vi "GBD_Header.vi"(7 "Head":string, 8 "Save?":bool, 9 "Mode":enum16{"Open", "Close", "Index"}(ring), 10 "Cvt_Mode":bool, 11 "File[]":path[](array[path])) -> (0 "error out":errorcluster, 1 "ActiveCH":i32, 2 "List":string[][](array[string]), 3 "Param":T1={"File"=[refnum], "Idx"=[], "dT"=0.5, "Hd"=4096, "Rd"=14, "Start"=[timestamp(3519879471 s since 1904-01-01)], "Trig"=[timestamp(3519879472 s since 1904-01-01)], "Stop"=[timestamp(3519940623 s since 1904-01-01)], "FirstPos"=[], "Count"=[120609], "Color"=[27836, 4765252, 11010216, 14712848], "Label"=["CH1", "CH2", "CH3", "CH4"], "INP"=["CH1", "CH2", "CH3", "CH4"], "H"=[5.0, 5.0, 5.0, 5.0], "L"=[-5.0, -5.0, -5.0, -5.0], "Fmt"=["%.;%+0.3f V", "%.;%+0.3f V", "%.;%+0.3f V", "%.;%+0.3f V"], "Unit"=["", "", "", ""], "SEL"=[0, 1, 2, 3], "Byte"=[-2, -2, -2, -2], "Pos"=[], "Bit"=[], "Flg"=[], "Gain"=[], "Offset"=[0.01, 0.01, 0.01, 0.01], "CH"=[0, 0, 0, 0], "Opt"={"Mode"=0, "TUNIT"=enum."CELS"}, "TYPE"=enum."GBD", "Comp"=[], "Temp"=[]} caption="HEAD" {"FirstPos" format="%<%x %.3X>T"; "Stop" format="%<%x %.3X>T"; "Trig" format="%<%x %.3X>T"; "Start" format="%<%x %.3X>T"}, 4 "Linkcheck":string[](array[string])=["Sampling", "Start", "Trigger", "Stop", "Count"])   [LabVIEW 2017]
uses:
  Amp_Param.ctl
panel:
  in  "Info":string[](array[string])=["Sampling", "Start", "Trigger", "Stop", "Count"]
  # "ALL"
  # "GBD"
  # "CSV"
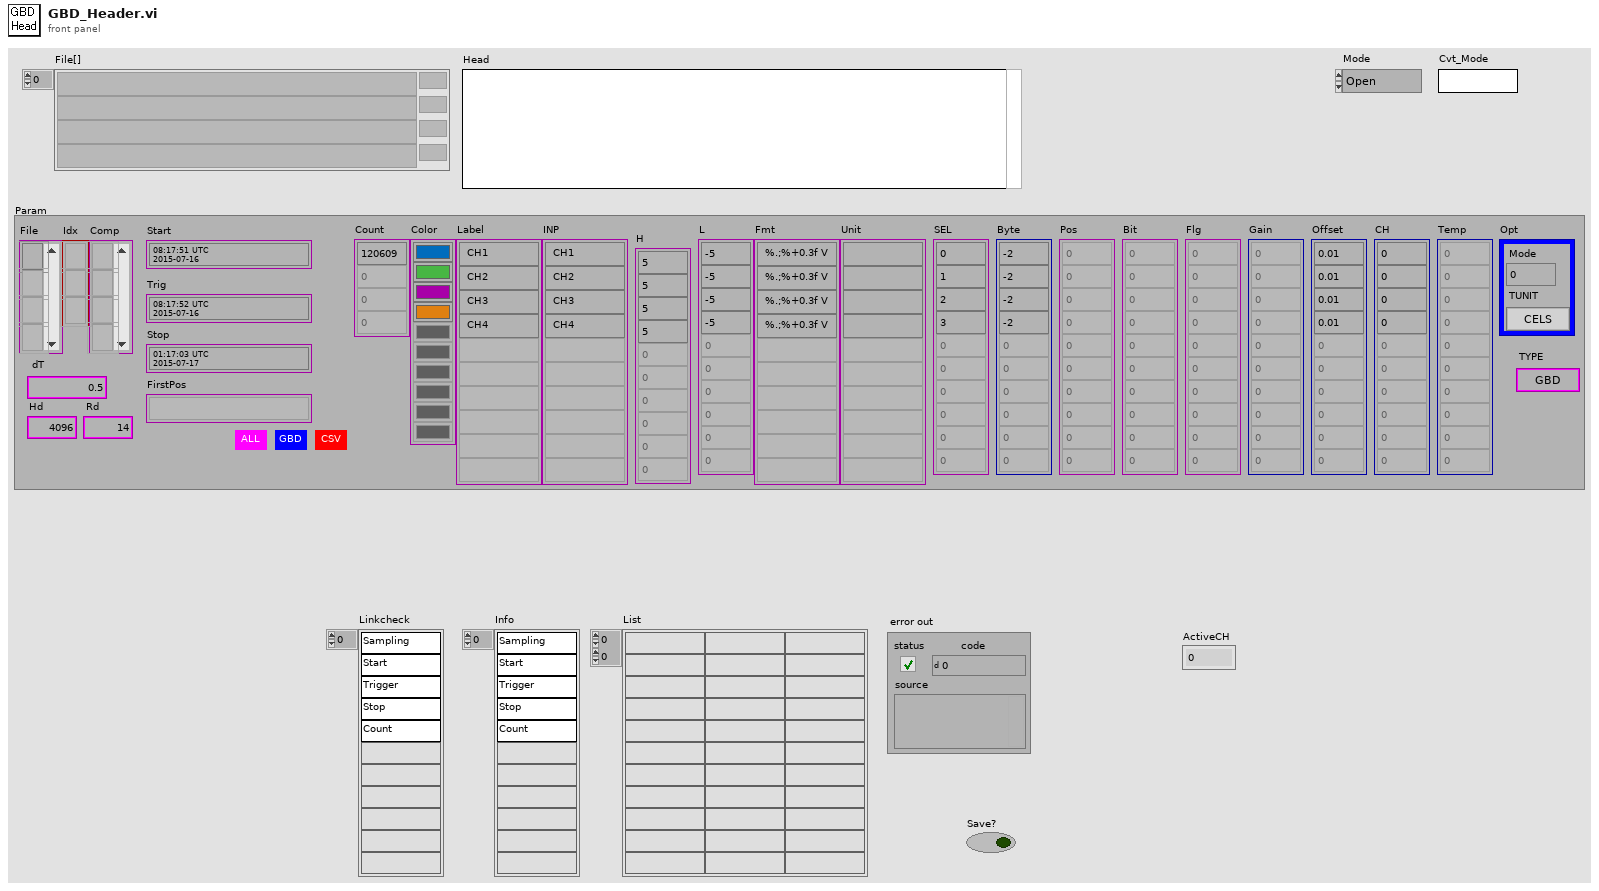
[diagram p1: front panel]
types:
  T1 = typedef "Amp_Param.ctl" = cluster{"File":refnum<file>[], "Idx":refnum<file>[], "dT":dbl, "Hd":i32, "Rd":i32, "Start":timestamp[], "Trig":timestamp[], "Stop":timestamp[], "FirstPos":timestamp[], "Count":i64[], "Color":u32[], "Label":string[], "INP":string[], "H":dbl[], "L":dbl[], "Fmt":string[], "Unit":string[], "SEL":i32[], "Byte":i32[], "Pos":i32[], "Bit":i32[], "Flg":i32[], "Gain":dbl[], "Offset":dbl[], "CH":i32[], "Opt":cluster{"Mode":i32, "TUNIT":enum16{"CELS", "FAHR"}}, "TYPE":enum16{"GBD", "CSV"}, "Comp":refnum<file>[], "Temp":i32[]}
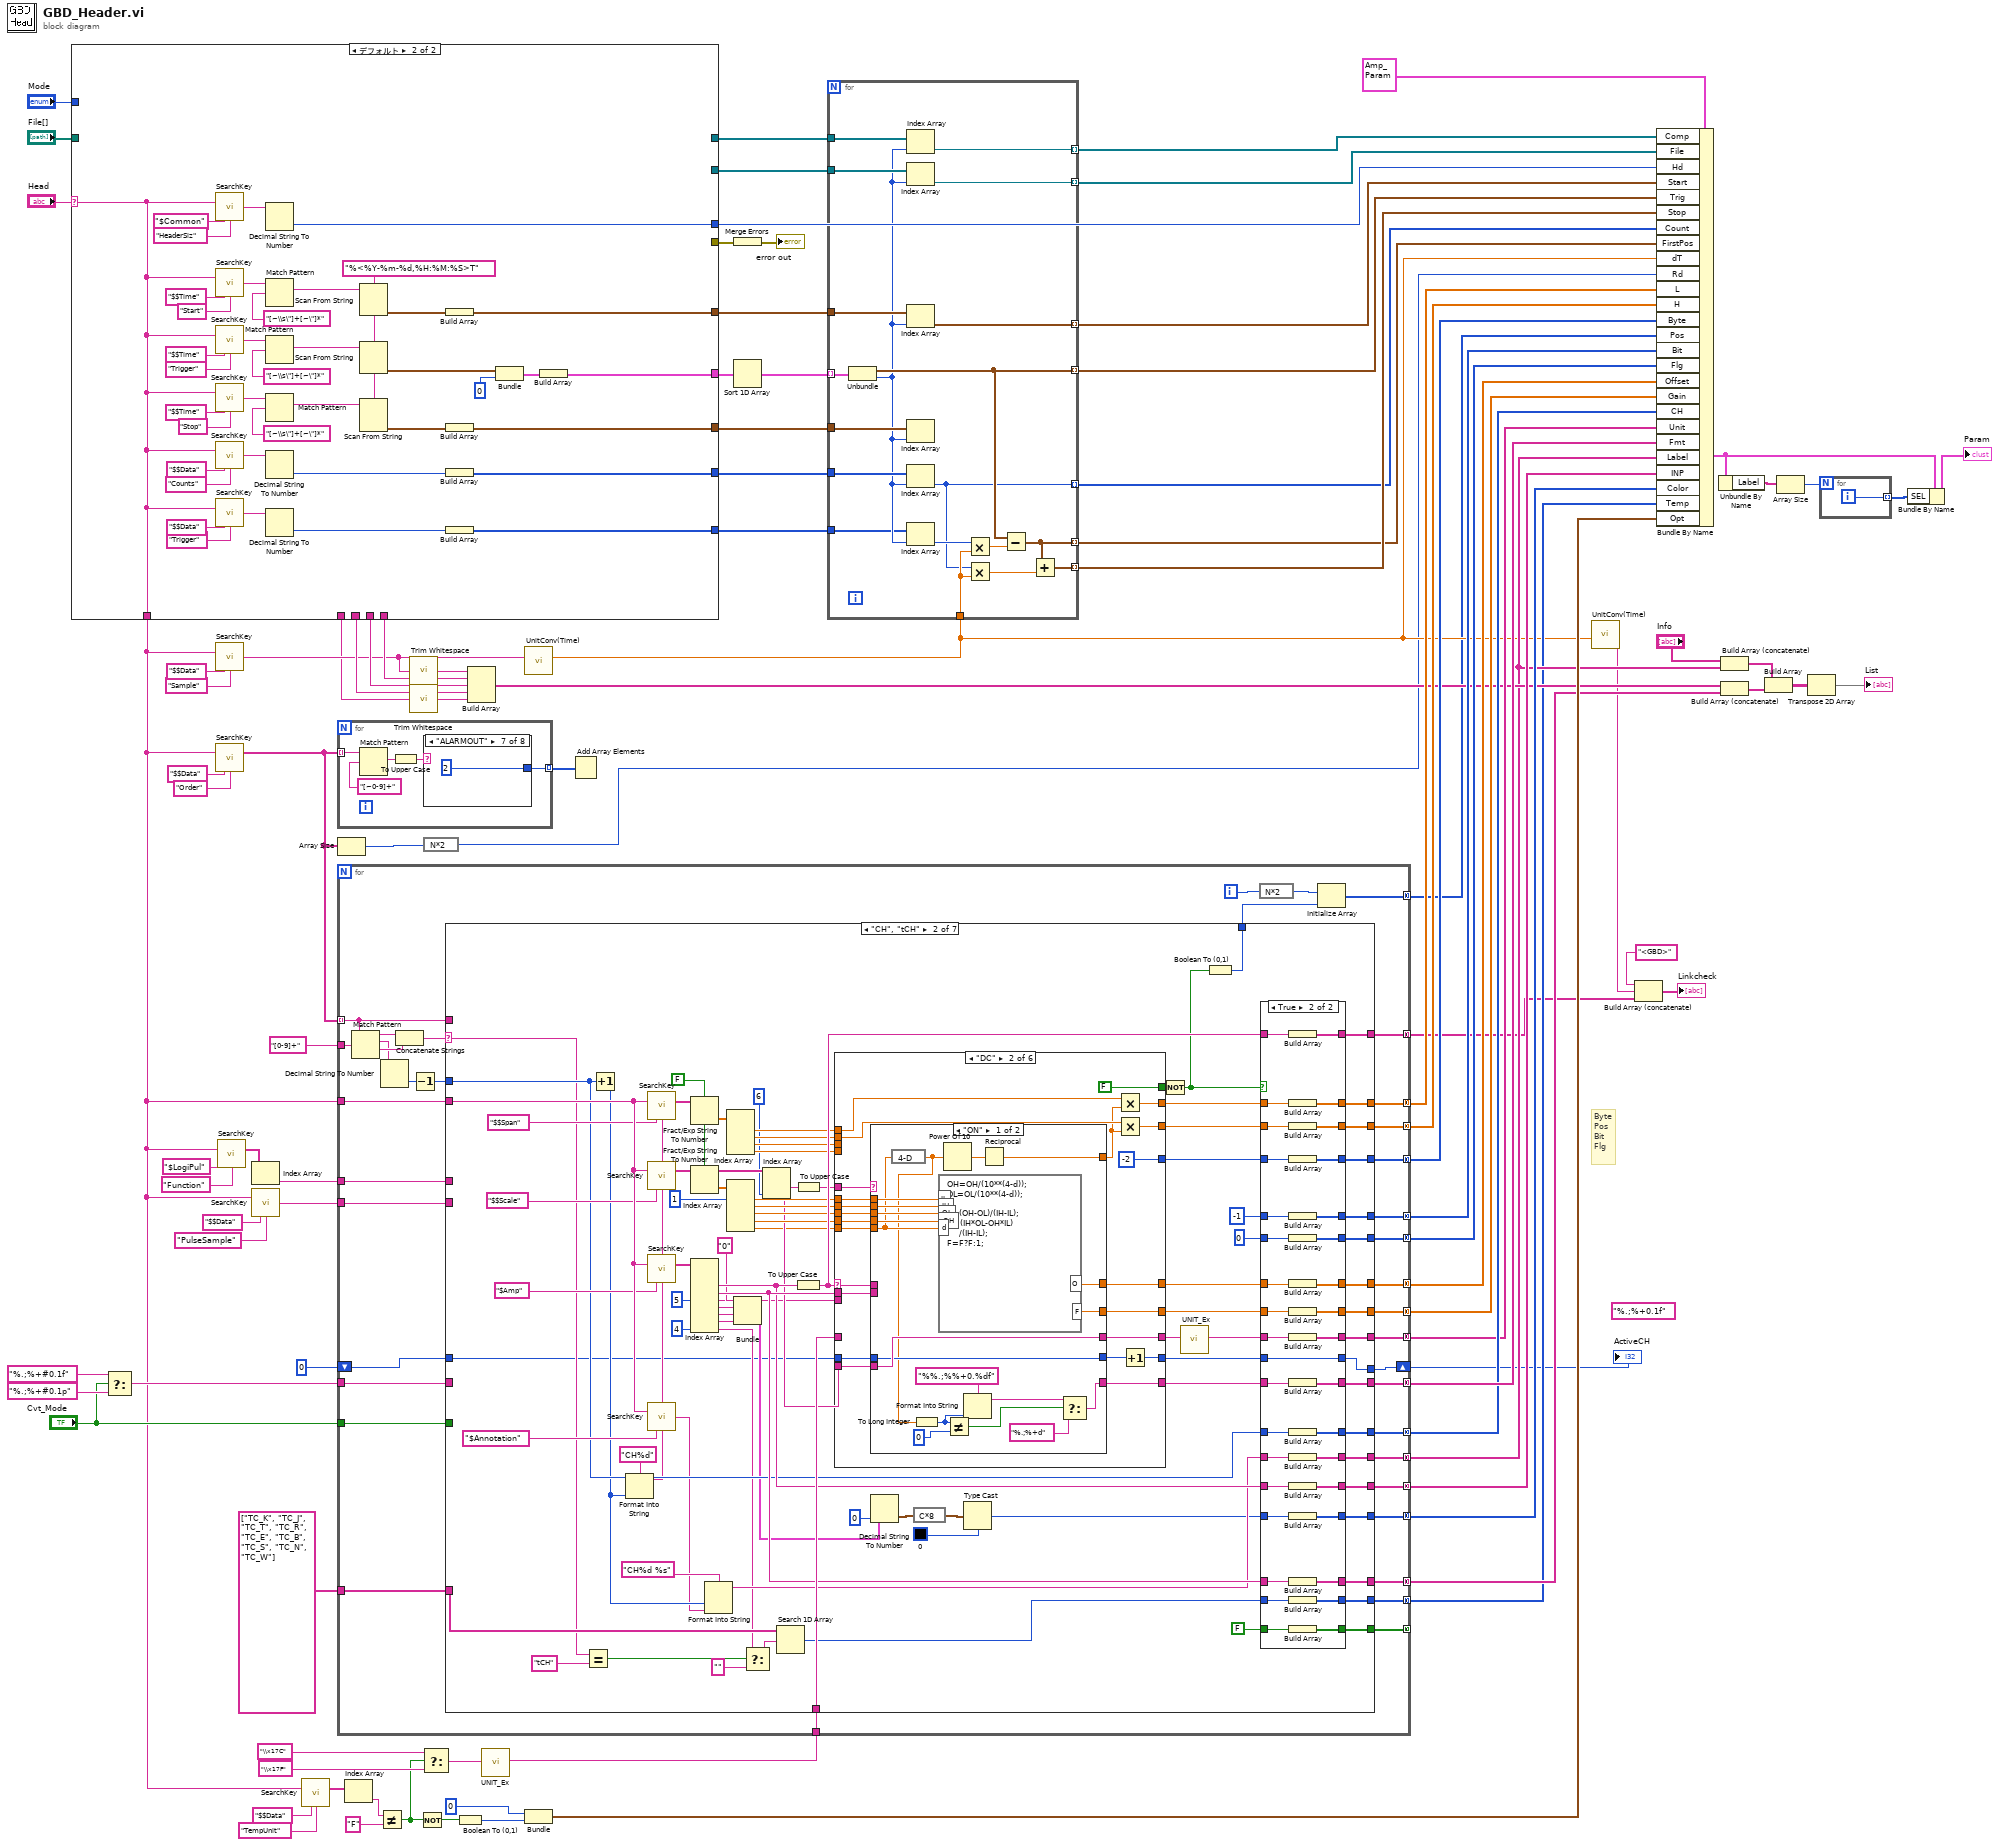
[diagram p0: block diagram]
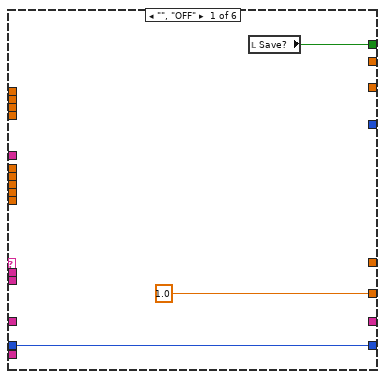
[diagram p4: hidden frame]
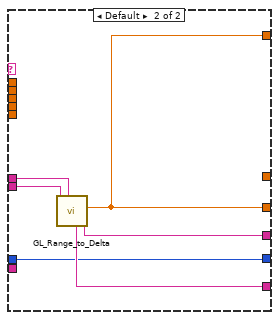
[diagram p5: hidden frame]
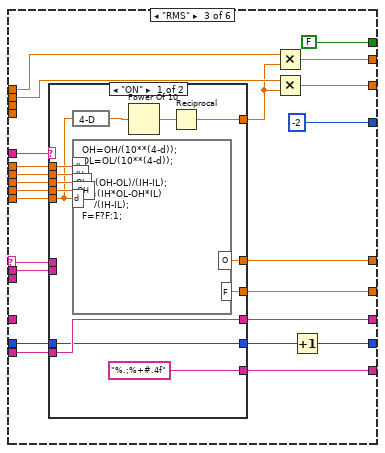
[diagram p6: hidden frame]
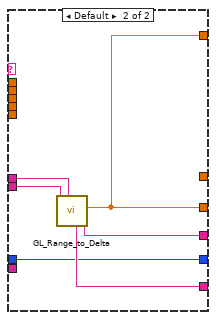
[diagram p7: hidden frame]
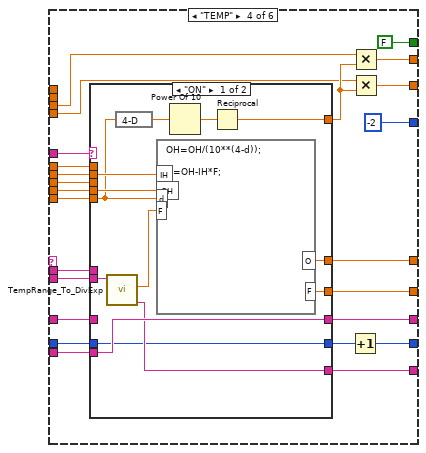
[diagram p8: hidden frame]
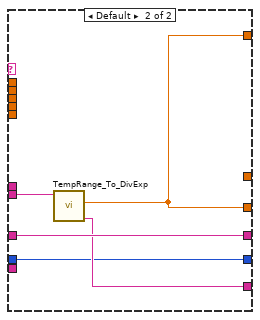
[diagram p9: hidden frame]
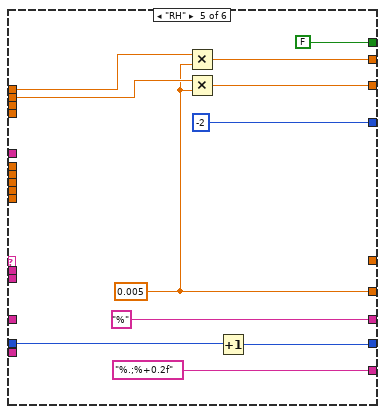
[diagram p10: hidden frame]
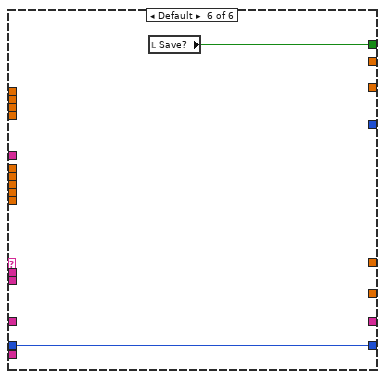
[diagram p11: hidden frame]
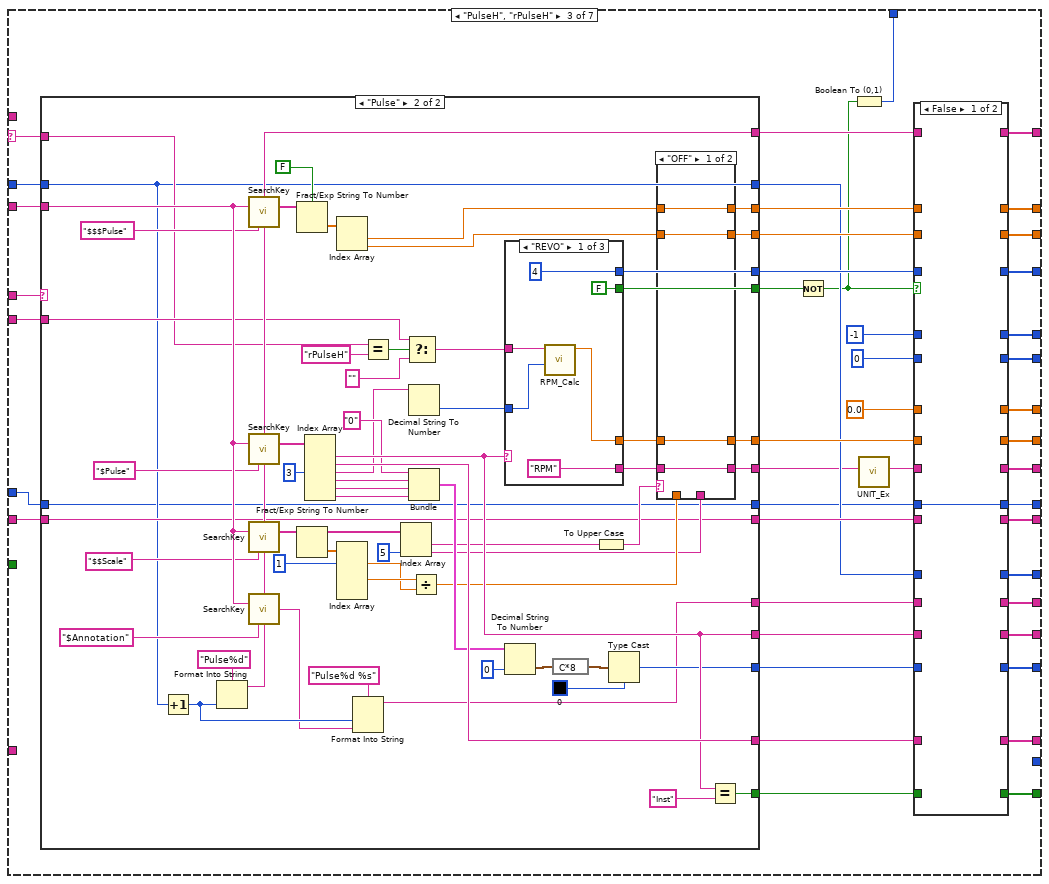
[diagram p12: hidden frame]
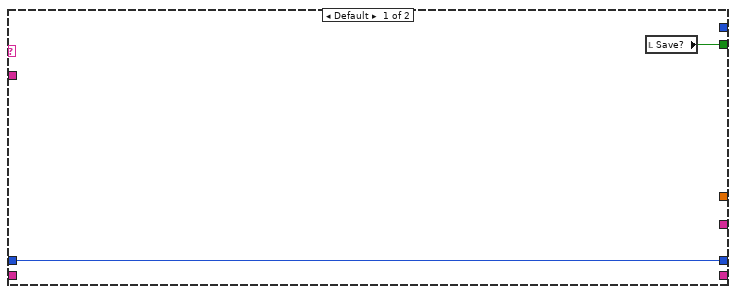
[diagram p13: hidden frame]
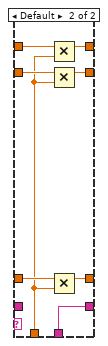
[diagram p14: hidden frame]
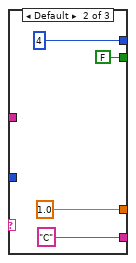
[diagram p15: hidden frame]
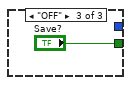
[diagram p16: hidden frame]
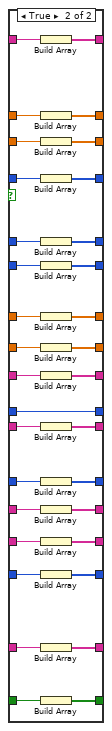
[diagram p17: hidden frame]
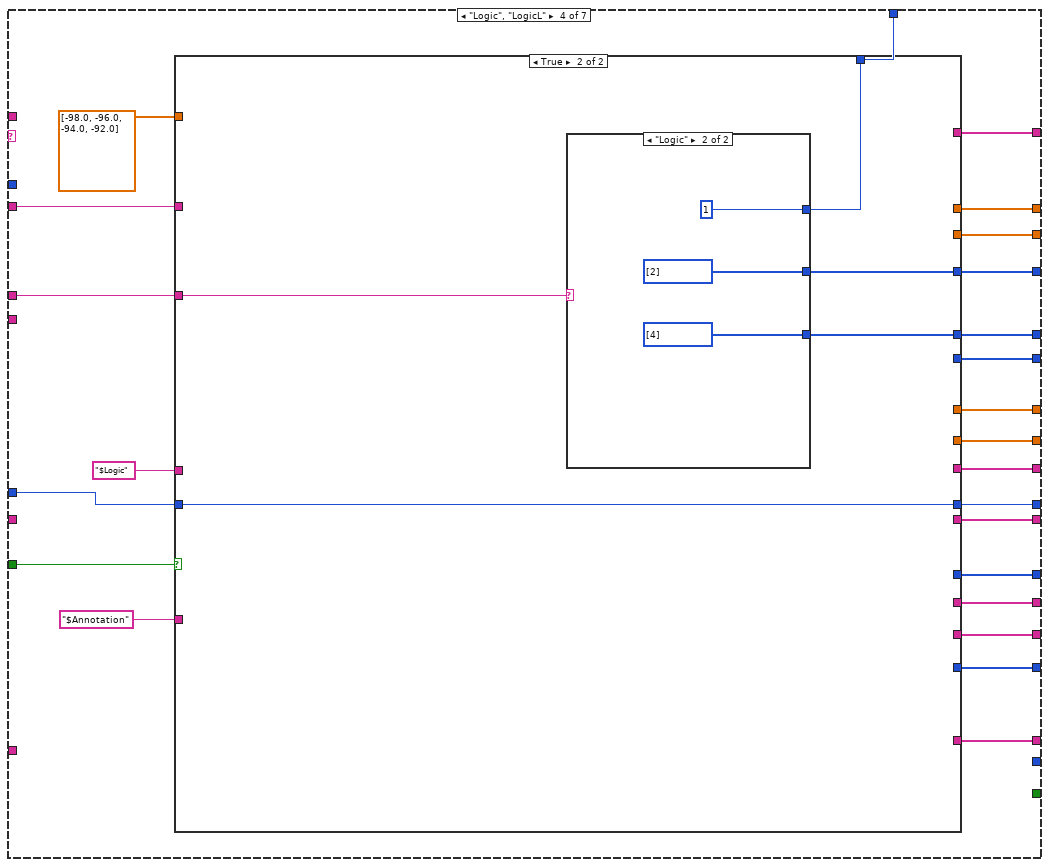
[diagram p18: hidden frame]
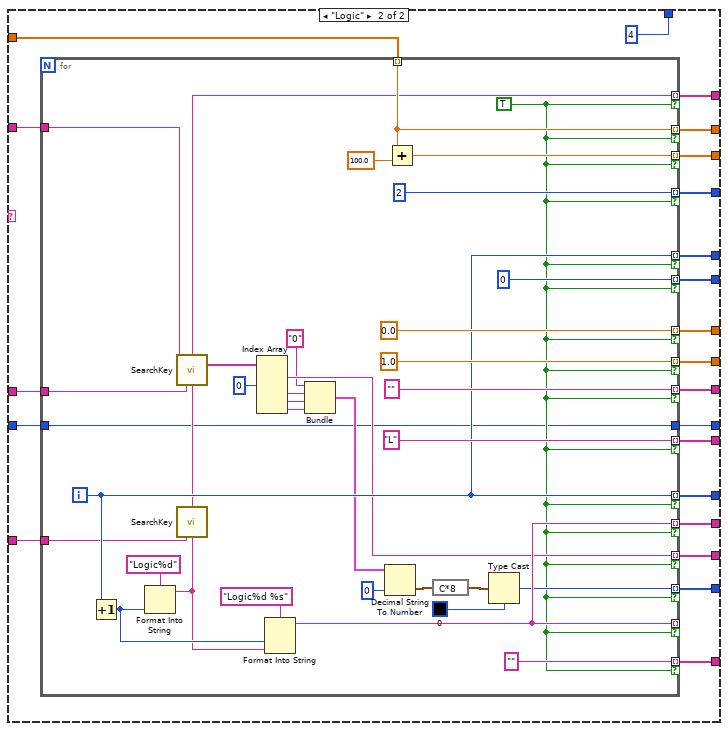
[diagram p20: hidden frame]
diagram:
  (unwired) "%.;%+0.1f" ("format string")
  # "Byte\nPos\nBit\nFlg"
  n1 = case shown="デフォルト" "Head" {
    selector: "Head" -> [_ w172]
    tunnel: [w115 _] -> w70
    tunnel: [w114 w185] -> w96
    tunnel: [w113 w172] -> w7
    tunnel: [w111 w209] -> w68
    tunnel: "File[]" -> [w112 _]
    tunnel: [w109 w182] -> w71
    tunnel: [w110 w181] -> w69
    tunnel: [w108 _] -> w77
    tunnel: [w107 _] -> w29
    tunnel: [w106 _] -> w76
    tunnel: "Mode" -> [w105 _]
    tunnel: [w104 w177] -> w74
    tunnel: [w103 _] -> w61
    tunnel: [w102 _] -> w39
    tunnel: [w101 w171] -> w27
    tunnel: [w100 _] -> w20
    frame "" {
      n2 = for {
        tunnel: [w121] -> w113
        tunnel: w112 -> [w130] mode=indexing
        tunnel: [w135] -> w115 mode=indexing
        tunnel: [w128] -> w114
        tunnel: [w148] -> w111 mode=indexing
        tunnel: [w139] -> w110 mode=indexing
        tunnel: [w138] -> w109 mode=indexing
        tunnel: [w125] -> w108
        tunnel: [w124] -> w107
        tunnel: [w126] -> w106
        tunnel: w105 -> [w134]
        tunnel: [w132] -> w104 mode=indexing
        tunnel: [w129] -> w103 mode=indexing
        tunnel: [w127] -> w102
        tunnel: [w120] -> w101 mode=indexing
        tunnel: [w117] -> w100 mode=indexing
        i -> [w133]
        w137 = "%<%Y-%m-%d,%H:%M:%S>T" ("format string")
        n3 = Open/Create/Replace File(file path (use dialog)=w130) -> (refnum out=w156:refnum<file>, error out=w155:errorcluster)  [unwired: 1 in, 5 out]
        n4 = Read from Binary File(8:w155, 10:1024 ("count"), 11:w156) -> (0:w116:errorcluster, 2:w118:string, 3:w162:refnum<file>)  [unwired: 4 out]
        n5 = call "SearchKey.vi"("In"=w118, "KEY1"="$Common", "KEY2"="HeaderSiz") -> ("String"=w159:string)  [unwired: 12 out]
        n6 = Set File Position(refnum=w162, from (0:start)=enum16{"start", "end", "current"}."start" ("pos mode (0:2)"), error in=w116) -> (refnum out=w158:refnum<file>, error out=w157:errorcluster)  [unwired: 1 out]
        n7 = Decimal String To Number(string=w159) -> (number=w128:i32)  [unwired: 3 out]
        n8 = Read from Binary File(8:w157, 10:w128, 11:w158) -> (0:w117:errorcluster, 2:w121:string, 3:w136:refnum<file>)  [unwired: 4 out]
        n9 = call "SearchKey.vi"("In"=w121, "KEY1"="$$Time", "KEY2"="Start") -> ("String"=w147:string)  [unwired: 12 out]
        n10 = call "SearchKey.vi"("In"=w121, "KEY1"="$$Time", "KEY2"="Trigger") -> ("String"=w149:string)  [unwired: 12 out]
        n11 = call "SearchKey.vi"("In"=w121, "KEY1"="$$Time", "KEY2"="Stop") -> ("String"=w140:string)  [unwired: 12 out]
        n12 = call "SearchKey.vi"("In"=w121, "KEY1"="$$Data", "KEY2"="Counts") -> ("String"=w124:string)  [unwired: 12 out]
        n13 = call "SearchKey.vi"("In"=w121, "KEY1"="$$Data", "KEY2"="Trigger") -> ("String"=w123:string)  [unwired: 12 out]
        n14 = Match Pattern(string=w147, regular expression="[~\\s\"]+[~\"]*") -> (match substring=w127:string)  [unwired: 4 out]
        n15 = Match Pattern(string=w149, regular expression="[~\\s\"]+[~\"]*") -> (match substring=w126:string)  [unwired: 4 out]
        n16 = Match Pattern(string=w140, regular expression="[~\\s\"]+[~\"]*") -> (match substring=w125:string)  [unwired: 4 out]
        n17 = Decimal String To Number(string=w123) -> (number=w120:i32)  [unwired: 3 out]
        n18 = Scan From String(format string=w137, input string=w127) -> (output 1=w138:timestamp)  [unwired: 3 in, 3 out]
        n19 = Scan From String(format string=w137, input string=w126) -> (output 1=w131:timestamp)  [unwired: 3 in, 3 out]
        n20 = Scan From String(format string=w137, input string=w125) -> (output 1=w139:timestamp)  [unwired: 3 in, 3 out]
        n21 = Decimal String To Number(string=w124) -> (number=w148:i32)  [unwired: 3 out]
        n22 = case shown="デフォルト" w134 {
          tunnel: w136 -> [w165 w170]
          tunnel: [_ w170] -> w135
          tunnel: w130 -> [_ w169]
          tunnel: [_ w167] -> w129
          tunnel: w128 -> [_ w166]
          frame "Close" {
            n23 = Close File(refnum=w165) -> ()  [unwired: 1 in, 2 out]
          }
          frame Default {
            n24 = Open/Create/Replace File(file path (use dialog)=w169) -> (refnum out=w168:refnum<file>)  [unwired: 1 in, 6 out]
            n25 = Set File Position(offset (in bytes) (0)=w166, refnum=w168) -> (refnum out=w167:refnum<file>)  [unwired: 2 in, 1 out]
          }
        }
        n26 = Bundle(w131, w133) -> (w132:cluster{timestamp, i32})  [unwired: 1 in]
      }
    }
    frame Default {
      w186 = "%<%Y-%m-%d,%H:%M:%S>T" ("format string")
      n27 = call "SearchKey.vi"("In"=w172, "KEY1"="$Common", "KEY2"="HeaderSiz") -> ("String"=w206:string)  [unwired: 12 out]
      n28 = call "SearchKey.vi"("In"=w172, "KEY1"="$$Time", "KEY2"="Start") -> ("String"=w196:string)  [unwired: 12 out]
      n29 = call "SearchKey.vi"("In"=w172, "KEY1"="$$Time", "KEY2"="Trigger") -> ("String"=w199:string)  [unwired: 12 out]
      n30 = call "SearchKey.vi"("In"=w172, "KEY1"="$$Time", "KEY2"="Stop") -> ("String"=w189:string)  [unwired: 12 out]
      n31 = call "SearchKey.vi"("In"=w172, "KEY1"="$$Data", "KEY2"="Counts") -> ("String"=w203:string)  [unwired: 12 out]
      n32 = call "SearchKey.vi"("In"=w172, "KEY1"="$$Data", "KEY2"="Trigger") -> ("String"=w175:string)  [unwired: 12 out]
      n33 = Decimal String To Number(string=w206) -> (number=w185:i32)  [unwired: 3 out]
      n34 = Match Pattern(string=w196, regular expression="[~\\s\"]+[~\"]*") -> (match substring=w197:string)  [unwired: 4 out]
      n35 = Match Pattern(string=w199, regular expression="[~\\s\"]+[~\"]*") -> (match substring=w198:string)  [unwired: 4 out]
      n36 = Match Pattern(string=w189, regular expression="[~\\s\"]+[~\"]*") -> (match substring=w188:string)  [unwired: 4 out]
      n37 = Decimal String To Number(string=w203) -> (number=w187:i32)  [unwired: 3 out]
      n38 = Decimal String To Number(string=w175) -> (number=w176:i32)  [unwired: 3 out]
      n39 = Scan From String(format string=w186, input string=w197) -> (output 1=w183:timestamp)  [unwired: 3 in, 3 out]
      n40 = Scan From String(format string=w186, input string=w198) -> (output 1=w180:timestamp)  [unwired: 3 in, 3 out]
      n41 = Scan From String(format string=w186, input string=w188) -> (output 1=w184:timestamp)  [unwired: 3 in, 3 out]
      n42 = Build Array(w183) -> (w182:timestamp[])
      n43 = Build Array(w184) -> (w181:timestamp[])
      n44 = Build Array(w187) -> (w209:i32[])
      n45 = Build Array(w176) -> (w171:i32[])
      n46 = Bundle(w180, 0) -> (w179:cluster{timestamp, i32})  [unwired: 1 in]
      n47 = Build Array(w179) -> (w177:cluster{timestamp, i32}[])
    }
  }
  n48 = Select(t="%.;%+#0.1f" ("format string"), s="Cvt_Mode", f="%.;%+#0.1p" ("format string")) -> (s? t:f=w23:string)
  n49 = call "SearchKey.vi"("In"=w7, "KEY1"="$$Data", "KEY2"="Sample") -> ("String"=w32:string)  [unwired: 12 out]
  n50 = call "SearchKey.vi"("In"=w7, "KEY1"="$$Data", "KEY2"="Order") -> ("Data"=w11:string[])  [unwired: 12 out]
  n51 = call "SearchKey.vi"("In"=w7, "KEY1"="$LogiPul", "KEY2"="Function") -> ("Data"=w48:string[])  [unwired: 12 out]
  n52 = Index Array(array=w48) -> (element=w4:string)  [unwired: 1 in]
  n53 = call "SearchKey.vi"("In"=w7, "KEY1"="$$Data", "KEY2"="PulseSample") -> ("String"=w12:string)  [unwired: 12 out]
  n54 = call "SearchKey.vi"("In"=w7, "KEY1"="$$Data", "KEY2"="TempUnit") -> ("Data"=w93:string[])  [unwired: 12 out]
  n55 = for {
    tunnel: w11 -> [w214] mode=indexing
    tunnel: [w211] -> w55 mode=indexing
    n56 = Match Pattern(string=w214, regular expression="[~0-9]+") -> (match substring=w213:string)  [unwired: 4 out]
    n57 = To Upper Case(1:w213) -> (0:w212:string)
    n58 = case shown="\"ALARMOUT\"" w212 {
      tunnel: [_ 2 ("element") 4 ("element") 2 ("element") 2 ("element") 2 ("element") 2 ("element") 2 ("element")] -> w211
      frame Default {
      }
      frame "CH" {
      }
      frame "HCH" {
      }
      frame "LOGIC" {
      }
      frame "ALARM" {
      }
      frame "ALARMLP" {
      }
      frame "ALARMOUT" {
      }
      frame "PULSE" {
      }
    }
  }
  n59 = Array Size(array=w11) -> (size(s)=w10:i32)
  n60 = Index Array(array=w93) -> (element=w87:string)  [unwired: 1 in]
  n61 = Not Equal?(x=w87, y="F") -> (x != y?=w59:bool)
  n62 = call <vilib>:"Trim Whitespace.vi"("string"=w32) -> ("trimmed string"=w31:string)  [unwired: 1 in]
  n63 = call <vilib>:"Trim Whitespace.vi"("string"=w29) -> ("trimmed string"=w30:string)  [unwired: 1 in]
  n64 = Not(x=w59) -> (.not. x?=w86:bool)
  n65 = Select(t="\\x17C" ("y"), s=w59, f="\\x17F" ("y")) -> (s? t:f=w84:string)
  n66 = expression code="N*2"(w10) -> (w9:i32)
  n67 = Boolean To (0,1)(Boolean=w86) -> (0, 1=w85:i16)
  n68 = Build Array(w31, w39, w76, w77, w30) -> (w41:string[])
  n69 = call "UNIT_Ex.vi"("In"=w84) -> ("Out"=w83:string)  [unwired: 10 out]
  n70 = for {
    tunnel: w7 -> [w259]
    tunnel: w83 -> [w258]
    tunnel: [w257] -> w54 mode=concatenating
    tunnel: [w256] -> w53 mode=concatenating
    tunnel: [w255] -> w81 mode=concatenating
    tunnel: [w254] -> w80 mode=concatenating
    tunnel: [w253] -> w79 mode=concatenating
    tunnel: [w252] -> w78 mode=concatenating
    tunnel: [w251] -> w37 mode=concatenating
    tunnel: [w250] -> w40 mode=concatenating
    tunnel: [w249] -> w63 mode=concatenating
    tunnel: [w248] -> w58 mode=concatenating
    tunnel: [w247] -> w57 mode=concatenating
    tunnel: [w246] -> w56 mode=concatenating
    tunnel: [w245] -> w51 mode=concatenating
    tunnel: [w244] -> w47 mode=concatenating
    tunnel: "Cvt_Mode" -> [w243]
    tunnel: [w242] -> w26 mode=concatenating
    tunnel: w23 -> [w241]
    tunnel: [w240] -> _ mode=concatenating
    tunnel: [w239] -> w18 mode=concatenating
    tunnel: w12 -> [w238]
    tunnel: w11 -> [w237] mode=indexing
    tunnel: "[0-9]+" ("KEY2") -> [w236]
    tunnel: [w227] -> w5 mode=concatenating
    tunnel: w4 -> [w230]
    tunnel: string[] ["TC_K", "TC_J", "TC_T", "TC_R", "TC_E", "TC_B", "TC_S", "TC_N", "TC_W"] ("1D array") -> [w225]
    shift-right: [w222] -> w2
    shift-left: 0 -> [w223]
    i -> [w224]
    n71 = Match Pattern(string=w237, regular expression=w236) -> (before substring=w235:string, match substring=w232:string, after substring=w233:string)  [unwired: 1 in, 1 out]
    n72 = Decimal String To Number(string=w232) -> (number=w231:i32)  [unwired: 2 in, 1 out]
    n73 = Concatenate Strings(w235, w233) -> (w234:string)
    n74 = Decrement(x=w231) -> (x-1=w229:i32)
    n75 = case shown="\"CH\", \"tCH\"" w234 {
      selector: w234 -> [_ w269 w553 _ _ _ _]
      tunnel: w259 -> [_ w351 w580 w710 w819 w860 _]
      tunnel: w258 -> [_ w350 _ _ _ _ _]
      tunnel: [_ w294 w566 w724 _ _ _] -> w257
      tunnel: [_ w293 w552 w723 _ _ _] -> w256
      tunnel: [_ w292 w565 w722 w817 w857 w920] -> w255
      tunnel: [_ w289 w562 w721 w822 w863 w919] -> w254
      tunnel: [_ w288 w561 w720 w821 w862 w918] -> w253
      tunnel: [_ w286 w559 w719 _ _ _] -> w252
      tunnel: [_ w284 w550 w718 _ _ _] -> w251
      tunnel: [_ w281 w555 w717 _ _ _] -> w250
      tunnel: [_ w283 w557 w716 _ _ _] -> w249
      tunnel: [_ w285 w558 w714 _ _ _] -> w248
      tunnel: [_ w282 w556 w713 _ _ _] -> w247
      tunnel: [_ w287 w560 w712 _ _ _] -> w246
      tunnel: [_ w291 w564 w711 w820 w861 w917] -> w245
      tunnel: [_ w290 w563 w709 w818 w859 w916] -> w244
      tunnel: w243 -> [_ _ _ w703 w815 w855 w914]
      tunnel: [_ w280 _ _ _ _ _] -> w242
      tunnel: w241 -> [_ _ w547 _ _ _ _]
      tunnel: [_ w279 w554 _ _ _ _] -> w240
      tunnel: [_ w295 w567 w706 _ _ _] -> w239
      tunnel: w238 -> [_ _ w568 _ _ _ _]
      tunnel: w237 -> [_ _ _ _ _ _ _]
      tunnel: w229 -> [_ w331 w545 _ _ _ _]
      tunnel: w230 -> [_ _ w543 w704 _ w858 _]
      tunnel: [_ w276 w541 w705 w816 w856 w915] -> w226
      tunnel: w225 -> [_ w275 _ _ _ _ _]
      tunnel: w223 -> [w260 w263 w538 w702 w814 w854 w913]
      tunnel: [w260 w261 w536 w701 w813 w854 w913] -> w222
      frame Default {
      }
      frame "CH", "tCH" {
        w296 = FALSE ("use system decimal point (T)")
        n76 = Equal?(x=w269, y="tCH") -> (x = y?=w268:bool)
        n77 = Increment(x=w331) -> (x+1=w321:i32)
        n78 = Format Into String(format string="CH%d" ("KEY1"), w321) -> (resulting string=w305:string)  [unwired: 2 in, 1 out]
        n79 = call "SearchKey.vi"("In"=w351, "KEY1"="$$Span", "KEY2"=w305) -> ("Data"=w327:string[])  [unwired: 12 out]
        n80 = call "SearchKey.vi"("In"=w351, "KEY1"="$$Scale", "KEY2"=w305) -> ("Data"=w308:string[])  [unwired: 12 out]
        n81 = call "SearchKey.vi"("In"=w351, "KEY1"="$Amp", "KEY2"=w305) -> ("Data"=w329:string[])  [unwired: 12 out]
        n82 = call "SearchKey.vi"("In"=w351, "KEY1"="$Annotation", "KEY2"=w305) -> ("String"=w320:string)  [unwired: 12 out]
        n83 = Fract/Exp String To Number(use system decimal point (T)=w296, string=w327) -> (number=w326:dbl[])  [unwired: 2 in, 1 out]
        n84 = Fract/Exp String To Number(use system decimal point (T)=w296, string=w308) -> (number=w309:dbl[])  [unwired: 2 in, 1 out]
        n85 = Index Array(array=w329, index #4=5 ("index"), index #8=4 ("index")) -> (element #2=w342:string, element #3=w343:string, element #4=w264:string, element #5=w319:string, element #6=w318:string, element #7=w311:string, element #8=w273:string)  [unwired: 6 in, 1 out]
        n86 = Format Into String(format string="CH%d %s" ("KEY1"), w321, w320) -> (resulting string=w341:string)  [unwired: 2 in, 1 out]
        n87 = Index Array(array=w326) -> (element #1=w325:dbl, element #2=w324:dbl, element #3=w323:dbl, element #4=w322:dbl)  [unwired: 4 in]
        n88 = Index Array(array=w309, index #1=1 ("index")) -> (element #1=w304:dbl, element #2=w303:dbl, element #3=w302:dbl, element #4=w301:dbl, element #5=w298:dbl)  [unwired: 4 in]
        n89 = Bundle("0", w319, w318, w311) -> (w312:cluster{string, string, string, string})  [unwired: 1 in]
        n90 = Select(t=w273, s=w268, f="") -> (s? t:f=w272:string)
        n91 = Index Array(array=w308, index #2=6 ("index")) -> (element #1=w307:string, element #2=w299:string)  [unwired: 1 in]
        n92 = Search 1D Array(1D array=w275, element=w272) -> (index of element=w271:i32)  [unwired: 1 in]
        n93 = To Upper Case(1:w342) -> (0:w332:string)
        n94 = To Upper Case(1:w307) -> (0:w297:string)
        n95 = case shown="\"DC\"" w332 {
          selector: w332 -> [_ w395 w443 _ _ _]
          tunnel: w343 -> [_ w408 w456 w501 _ _]
          tunnel: [1.0 w397 w445 w491 w527 _] -> w345
          tunnel: [_ w407 w455 w485 "%" ("Unit OUT") _] -> w266
          tunnel: w350 -> [_ _ _ w490 _ _]
          tunnel: [_ -2 -2 -2 -2 _] -> w347
          tunnel: w325 -> [_ w409 w457 _ w529 _]
          tunnel: w324 -> [_ w410 w458 _ w528 _]
          tunnel: w323 -> [_ _ _ w488 _ _]
          tunnel: w322 -> [_ _ _ w489 _ _]
          tunnel: [_ w412 w460 w503 w531 _] -> w349
          tunnel: [_ w411 w459 w502 w530 _] -> w348
          tunnel: [_ w406 w454 w500 "%.;%+0.2f" ("format string") _] -> w344
          tunnel: [w389 FALSE ("Save?") FALSE ("Save?") FALSE ("Save?") FALSE ("Save?") w535] -> w278
          tunnel: w304 -> [_ w403 w451 w497 _ _]
          tunnel: w303 -> [_ w402 w450 w496 _ _]
          tunnel: w302 -> [_ w401 w449 w495 _ _]
          tunnel: w301 -> [_ w400 w448 w494 _ _]
          tunnel: w298 -> [_ w399 w447 w493 _ _]
          tunnel: w297 -> [_ w405 w453 w499 _ _]
          tunnel: [_ w404 w452 w498 _ _] -> w346
          tunnel: w299 -> [_ w396 w444 w487 _ _]
          tunnel: w264 -> [_ _ _ w484 _ _]
          tunnel: [w388 w393 w441 w481 w523 w534] -> w262
          tunnel: w263 -> [w388 w391 w439 w483 w524 w534]
          frame "", "OFF" {
            n96 = local read "Save?"() -> (w389:bool)
          }
          frame "DC" {
            n97 = case shown="\"ON\"" w405 {
              tunnel: w408 -> [_ w438]
              tunnel: [w432 w435] -> w397
              tunnel: [w426 w437] -> w407
              tunnel: [w417 w436] -> w406
              tunnel: [w431 _] -> w404
              tunnel: w403 -> [w430 _]
              tunnel: w402 -> [w429 _]
              tunnel: w401 -> [w428 _]
              tunnel: w400 -> [w427 _]
              tunnel: w399 -> [w423 _]
              tunnel: [w424 w435] -> w398
              tunnel: w396 -> [w426 _]
              tunnel: w395 -> [_ w434]
              tunnel: [w422 w433] -> w392
              tunnel: w391 -> [w422 w433]
              frame "ON" {
                n98 = expression code="4-D"(w423) -> (w415:dbl)
                n99 = To Long Integer(number=w415) -> (32bit integer=w414:i32)
                n100 = formula code="OH=OH/(10**(4-d));\nOL=OL/(10**(4-d));\n\nF=(OH-OL)/(IH-IL);\nO=(IH*OL-OH*IL)\n    /(IH-IL);\nF=F?F:1;"("IL"=w430, "IH"=w429, "OL"=w428, "OH"=w427, "d"=w423) -> ("O"=w431:dbl, "F"=w432:dbl)
                n101 = Power Of 10(x=w415) -> (10^x=w425:dbl)
                n102 = Not Equal?(x=w414, y=0) -> (x != y?=w420:bool)
                n103 = Format Into String(format string="%%.;%%+0.%df", w414) -> (resulting string=w419:string)  [unwired: 2 in, 1 out]
                n104 = Reciprocal(x=w425) -> (1/x=w424:dbl)
                n105 = Select(t=w419, s=w420, f="%.;%+d" ("format string")) -> (s? t:f=w417:string)
              }
              frame Default {
                n106 = call "GL_Range_to_Delta.vi"("Input"=w434, "Range"=w438) -> ("Unit"=w437:string, "delta"=w435:dbl, "Fmt"=w436:string)  [unwired: 5 in]
              }
            }
            n107 = Multiply(x=w409, y=w398) -> (x*y=w412:dbl)
            n108 = Multiply(x=w410, y=w398) -> (x*y=w411:dbl)
            n109 = Increment(x=w392) -> (x+1=w393:i32)
          }
          frame "RMS" {
            n110 = case shown="\"ON\"" w453 {
              tunnel: w456 -> [_ w480]
              tunnel: [w474 w477] -> w445
              tunnel: [w467 w479] -> w455
              tunnel: ["%.;%+#.4f" ("Fmt") w478] -> w454
              tunnel: [w473 _] -> w452
              tunnel: w451 -> [w472 _]
              tunnel: w450 -> [w471 _]
              tunnel: w449 -> [w470 _]
              tunnel: w448 -> [w469 _]
              tunnel: w447 -> [w464 _]
              tunnel: [w463 w477] -> w446
              tunnel: w444 -> [w467 _]
              tunnel: w443 -> [_ w476]
              tunnel: [w462 w475] -> w440
              tunnel: w439 -> [w462 w475]
              frame "ON" {
                n111 = expression code="4-D"(w464) -> (w465:dbl)
                n112 = formula code="OH=OH/(10**(4-d));\nOL=OL/(10**(4-d));\n\nF=(OH-OL)/(IH-IL);\nO=(IH*OL-OH*IL)\n    /(IH-IL);\nF=F?F:1;"("IL"=w472, "IH"=w471, "OL"=w470, "OH"=w469, "d"=w464) -> ("O"=w473:dbl, "F"=w474:dbl)
                n113 = Power Of 10(x=w465) -> (10^x=w466:dbl)
                n114 = Reciprocal(x=w466) -> (1/x=w463:dbl)
              }
              frame Default {
                n115 = call "GL_Range_to_Delta.vi"("Input"=w476, "Range"=w480) -> ("Unit"=w479:string, "delta"=w477:dbl, "Fmt"=w478:string)  [unwired: 5 in]
              }
            }
            n116 = Multiply(x=w457, y=w446) -> (x*y=w460:dbl)
            n117 = Multiply(x=w458, y=w446) -> (x*y=w459:dbl)
            n118 = Increment(x=w440) -> (x+1=w441:i32)
          }
          frame "TEMP" {
            n119 = case shown="\"ON\"" w499 {
              tunnel: w501 -> [_ _]
              tunnel: [w517 w520] -> w491
              tunnel: [w511 w522] -> w485
              tunnel: [w506 w519] -> w500
              tunnel: [w516 _] -> w498
              tunnel: w497 -> [_ _]
              tunnel: w496 -> [w514 _]
              tunnel: w495 -> [_ _]
              tunnel: w494 -> [w515 _]
              tunnel: w493 -> [w510 _]
              tunnel: [w512 w520] -> w492
              tunnel: w490 -> [_ w522]
              tunnel: w487 -> [w511 _]
              tunnel: w484 -> [w507 w521]
              tunnel: w483 -> [w505 w518]
              tunnel: [w505 w518] -> w482
              frame "ON" {
                n120 = call "TempRange_To_DivExp.vi"("Range"=w507) -> ("Exp"=w506:string, "Div"=w508:dbl)  [unwired: 8 in]
                n121 = expression code="4-D"(w510) -> (w509:dbl)
                n122 = formula code="OH=OH/(10**(4-d));\n\nO=OH-IH*F;"("IH"=w514, "OH"=w515, "d"=w510, "F"=w508) -> ("O"=w516:dbl, "F"=w517:dbl)
                n123 = Power Of 10(x=w509) -> (10^x=w513:dbl)
                n124 = Reciprocal(x=w513) -> (1/x=w512:dbl)
              }
              frame Default {
                n125 = call "TempRange_To_DivExp.vi"("Range"=w521) -> ("Exp"=w519:string, "Div"=w520:dbl)  [unwired: 8 in]
              }
            }
            n126 = Increment(x=w482) -> (x+1=w481:i32)
            n127 = Multiply(x=w488, y=w492) -> (x*y=w503:dbl)
            n128 = Multiply(x=w489, y=w492) -> (x*y=w502:dbl)
          }
          frame "RH" {
            w527 = 0.005
            n129 = Multiply(x=w529, y=w527) -> (x*y=w531:dbl)
            n130 = Multiply(x=w528, y=w527) -> (x*y=w530:dbl)
            n131 = Increment(x=w524) -> (x+1=w523:i32)
          }
          frame Default {
            n132 = local read "Save?"() -> (w535:bool)
          }
        }
        n133 = Decimal String To Number(string=w312, default (0L)=u8 0 ("index")) -> (number=w315:cluster{u8, u8, u8, u8})  [unwired: 1 in, 1 out]
        n134 = expression code="C*8"(w315) -> (w313:cluster{u8, u8, u8, u8})
        n135 = Type Cast(type=u32 0 ("Color"), x=w313) -> (*(type *) &x=w338:u32)
        n136 = Not(x=w278) -> (.not. x?=w277:bool)
        n137 = call "UNIT_Ex.vi"("In"=w266) -> ("Out"=w265:string)  [unwired: 10 out]
        n138 = Boolean To (0,1)(Boolean=w277) -> (0, 1=w276:i16)
        n139 = case shown="TRUE" w277 {
          tunnel: w349 -> [_ w387]
          tunnel: w348 -> [_ w386]
          tunnel: w347 -> [_ w385]
          tunnel: w346 -> [_ w384]
          tunnel: w345 -> [_ w383]
          tunnel: w344 -> [_ w382]
          tunnel: w343 -> [_ w381]
          tunnel: w342 -> [_ w380]
          tunnel: w341 -> [_ w379]
          tunnel: w338 -> [_ w378]
          tunnel: w265 -> [_ w377]
          tunnel: -1 -> [_ w376]
          tunnel: 0 -> [_ w375]
          tunnel: w271 -> [_ w374]
          tunnel: FALSE -> [_ w373]
          tunnel: w332 -> [_ w372]
          tunnel: w331 -> [_ w371]
          tunnel: [_ w370] -> w295
          tunnel: [_ w369] -> w294
          tunnel: [_ w368] -> w293
          tunnel: [_ w367] -> w292
          tunnel: [_ w366] -> w291
          tunnel: [_ w365] -> w290
          tunnel: [_ w364] -> w289
          tunnel: [_ w363] -> w288
          tunnel: [_ w362] -> w287
          tunnel: [_ w361] -> w286
          tunnel: [_ w360] -> w285
          tunnel: [_ w359] -> w284
          tunnel: [_ w358] -> w283
          tunnel: [_ w357] -> w282
          tunnel: [_ w356] -> w281
          tunnel: [_ w355] -> w280
          tunnel: [_ w354] -> w279
          tunnel: w262 -> [w352 w353]
          tunnel: [w352 w353] -> w261
          frame False {
          }
          frame True {
            n140 = Build Array(w372) -> (w370:string[])
            n141 = Build Array(w387) -> (w369:dbl[])
            n142 = Build Array(w386) -> (w368:dbl[])
            n143 = Build Array(w385) -> (w367:i32[])
            n144 = Build Array(w376) -> (w366:i32[])
            n145 = Build Array(w375) -> (w365:i32[])
            n146 = Build Array(w384) -> (w364:dbl[])
            n147 = Build Array(w383) -> (w363:dbl[])
            n148 = Build Array(w377) -> (w362:string[])
            n149 = Build Array(w382) -> (w361:string[])
            n150 = Build Array(w371) -> (w360:i32[])
            n151 = Build Array(w379) -> (w359:string[])
            n152 = Build Array(w380) -> (w358:string[])
            n153 = Build Array(w378) -> (w357:u32[])
            n154 = Build Array(w381) -> (w356:string[])
            n155 = Build Array(w374) -> (w355:i32[])
            n156 = Build Array(w373) -> (w354:bool[])
          }
        }
      }
      frame "PulseH", "rPulseH" {
        n157 = case shown="\"Pulse\"" w543 {
          tunnel: w580 -> [_ w643]
          tunnel: [_ w642] -> w579
          tunnel: [_ w641] -> w578
          tunnel: [_ w640] -> w576
          tunnel: [_ w639] -> w575
          tunnel: [_ w638] -> w574
          tunnel: [_ w635] -> w573
          tunnel: [_ w634] -> w540
          tunnel: [_ w632] -> w570
          tunnel: [_ w631] -> w569
          tunnel: w568 -> [_ w630]
          tunnel: w545 -> [_ w584]
          tunnel: w553 -> [_ w590]
          tunnel: [_ w588] -> w551
          tunnel: [_ w587] -> w549
          tunnel: [w582 w586] -> w548
          tunnel: w547 -> [_ w585]
          tunnel: [_ w585] -> w546
          tunnel: [_ w584] -> w544
          tunnel: w538 -> [w581 w583]
          tunnel: [w581 w583] -> w537
          frame Default {
            n158 = local read "Save?"() -> (w582:bool)
          }
          frame "Pulse" {
            n159 = Increment(x=w584) -> (x+1=w623:i32)
            n160 = Format Into String(format string="Pulse%d" ("KEY1"), w623) -> (resulting string=w631:string)  [unwired: 2 in, 1 out]
            n161 = call "SearchKey.vi"("In"=w643, "KEY1"="$$$Pulse", "KEY2"=w631) -> ("Data"=w625:string[])  [unwired: 12 out]
            n162 = call "SearchKey.vi"("In"=w643, "KEY1"="$Pulse", "KEY2"=w631) -> ("Data"=w627:string[])  [unwired: 12 out]
            n163 = call "SearchKey.vi"("In"=w643, "KEY1"="$$Scale", "KEY2"=w631) -> ("Data"=w599:string[])  [unwired: 12 out]
            n164 = call "SearchKey.vi"("In"=w643, "KEY1"="$Annotation", "KEY2"=w631) -> ("String"=w613:string)  [unwired: 12 out]
            n165 = Fract/Exp String To Number(use system decimal point (T)=FALSE, string=w625) -> (number=w624:dbl[])  [unwired: 2 in, 1 out]
            n166 = Fract/Exp String To Number(string=w599) -> (number=w604:dbl[])  [unwired: 3 in, 1 out]
            n167 = Index Array(array=w627, index #3=3 ("index")) -> (element #1=w638:string, element #2=w639:string, element #3=w607:string, element #4=w618:string, element #5=w617:string, element #6=w616:string)  [unwired: 5 in]
            n168 = Index Array(array=w624) -> (element #1=w602:dbl, element #2=w603:dbl)  [unwired: 2 in]
            n169 = Index Array(array=w604, index #1=1 ("index")) -> (element #1=w594:dbl, element #3=w595:dbl)  [unwired: 4 in, 3 out]
            n170 = Format Into String(format string="Pulse%d %s" ("KEY1"), w623, w613) -> (resulting string=w587:string)  [unwired: 2 in, 1 out]
            n171 = Equal?(x=w590, y="rPulseH") -> (x = y?=w591:bool)
            n172 = Index Array(array=w599, index #2=5 ("index")) -> (element #1=w597:string, element #2=w592:string)  [unwired: 1 in]
            n173 = Select(t=w630, s=w591, f="") -> (s? t:f=w609:string)
            n174 = Decimal String To Number(string=w607) -> (number=w606:i32)  [unwired: 2 in, 1 out]
            n175 = Bundle("0", w618, w617, w616) -> (w615:cluster{string, string, string, string})  [unwired: 1 in]
            n176 = Divide(x=w595, y=w594) -> (x/y=w593:dbl)
            n177 = case shown="\"REVO\"" w638 {
              tunnel: [4 4 _] -> w641
              tunnel: ["RPM" ("format string") "C" ("format string") _] -> w600
              tunnel: [FALSE ("Save?") FALSE ("Save?") "Save?"] -> w586
              tunnel: w609 -> [w659 _ _]
              tunnel: [w658 1.0 ("y") _] -> w601
              tunnel: w606 -> [w657 _ _]
              frame "REVO" {
                n178 = call "RPM_Calc.vi"("Round"=w657, "PulseSampling"=w659) -> ("delta"=w658:dbl)  [unwired: 8 in, 1 out]
              }
              frame Default {
              }
              frame "OFF" {
              }
            }
            n179 = Decimal String To Number(string=w615, default (0L)=u8 0 ("index")) -> (number=w621:cluster{u8, u8, u8, u8})  [unwired: 1 in, 1 out]
            n180 = expression code="C*8"(w621) -> (w619:cluster{u8, u8, u8, u8})
            n181 = To Upper Case(1:w597) -> (0:w596:string)
            n182 = Type Cast(type=u32 0 ("Color"), x=w619) -> (*(type *) &x=w635:u32)
            n183 = case shown="\"OFF\"" w596 {
              tunnel: w603 -> [w646 w652]
              tunnel: w602 -> [w647 w653]
              tunnel: [w647 w651] -> w642
              tunnel: [w646 w650] -> w588
              tunnel: w601 -> [w645 w655]
              tunnel: [w645 w654] -> w640
              tunnel: w600 -> [w644 _]
              tunnel: [w644 w648] -> w634
              tunnel: w593 -> [_ w649]
              tunnel: w592 -> [_ w648]
              frame "OFF" {
              }
              frame Default {
                n184 = Multiply(x=w653, y=w649) -> (x*y=w651:dbl)
                n185 = Multiply(x=w652, y=w649) -> (x*y=w650:dbl)
                n186 = Multiply(x=w655, y=w649) -> (x*y=w654:dbl)
              }
            }
            n187 = Equal?(x=w638, y="Inst") -> (x = y?=w632:bool)
          }
        }
        n188 = Not(x=w548) -> (.not. x?=w542:bool)
        n189 = Boolean To (0,1)(Boolean=w542) -> (0, 1=w541:i16)
        n190 = call "UNIT_Ex.vi"("In"=w540) -> ("Out"=w539:string)  [unwired: 10 out]
        n191 = case shown="FALSE" w542 {
          tunnel: w579 -> [_ w700]
          tunnel: w578 -> [_ w699]
          tunnel: 0.0 -> [_ w698]
          tunnel: w576 -> [_ w697]
          tunnel: w575 -> [_ w696]
          tunnel: w574 -> [_ w695]
          tunnel: w573 -> [_ w694]
          tunnel: w539 -> [_ w693]
          tunnel: -1 -> [_ w692]
          tunnel: 0 -> [_ w691]
          tunnel: w546 -> [_ w690]
          tunnel: w570 -> [_ w689]
          tunnel: w569 -> [_ w688]
          tunnel: [_ w687] -> w567
          tunnel: [_ w686] -> w566
          tunnel: [_ w685] -> w565
          tunnel: [_ w684] -> w564
          tunnel: [_ w683] -> w563
          tunnel: [_ w682] -> w562
          tunnel: [_ w681] -> w561
          tunnel: [_ w680] -> w560
          tunnel: [_ w679] -> w559
          tunnel: [_ w678] -> w558
          tunnel: [_ w677] -> w557
          tunnel: [_ w676] -> w556
          tunnel: [_ w675] -> w555
          tunnel: [_ w674] -> w554
          tunnel: w544 -> [_ w673]
          tunnel: [_ w672] -> w552
          tunnel: w551 -> [_ w671]
          tunnel: [_ w670] -> w550
          tunnel: w549 -> [_ w669]
          tunnel: w537 -> [w667 w668]
          tunnel: [w667 w668] -> w536
          frame False {
          }
          frame True {
            n192 = Build Array(w688) -> (w687:string[])
            n193 = Build Array(w700) -> (w686:dbl[])
            n194 = Build Array(w671) -> (w672:dbl[])
            n195 = Build Array(w699) -> (w685:i32[])
            n196 = Build Array(w692) -> (w684:i32[])
            n197 = Build Array(w691) -> (w683:i32[])
            n198 = Build Array(w698) -> (w682:dbl[])
            n199 = Build Array(w697) -> (w681:dbl[])
            n200 = Build Array(w693) -> (w680:string[])
            n201 = Build Array(w690) -> (w679:string[])
            n202 = Build Array(w673) -> (w678:i32[])
            n203 = Build Array(w669) -> (w670:string[])
            n204 = Build Array(w695) -> (w677:string[])
            n205 = Build Array(w694) -> (w676:u32[])
            n206 = Build Array(w696) -> (w675:string[])
            n207 = Build Array(w689) -> (w674:bool[])
          }
        }
      }
      frame "Logic", "LogicL" {
        n208 = case shown="TRUE" w703 {
          tunnel: [w747 _] -> w724
          tunnel: [w746 _] -> w723
          tunnel: [w745 w808] -> w722
          tunnel: [w744 _] -> w721
          tunnel: [w743 _] -> w720
          tunnel: [w742 _] -> w719
          tunnel: [w741 _] -> w718
          tunnel: [w740 _] -> w717
          tunnel: [w739 _] -> w716
          tunnel: "$Logic" ("KEY1") -> [w738 _]
          tunnel: [w737 _] -> w714
          tunnel: [w736 _] -> w713
          tunnel: [w735 _] -> w712
          tunnel: [w734 w807] -> w711
          tunnel: w710 -> [w733 _]
          tunnel: [w732 _] -> w709
          tunnel: dbl[] [-98.0, -96.0, -94.0, -92.0] -> [w731 _]
          tunnel: "$Annotation" ("KEY1") -> [w730 _]
          tunnel: [w729 _] -> w706
          tunnel: [w728 w809] -> w705
          tunnel: w704 -> [w727 w806]
          tunnel: w702 -> [w726 w805]
          tunnel: [w725 w805] -> w701
          frame False {
            n209 = case shown="デフォルト" w727 {
              tunnel: [_ w770] -> w747
              tunnel: [_ w769] -> w746
              tunnel: [_ w768] -> w745
              tunnel: [_ w767] -> w744
              tunnel: [_ w766] -> w743
              tunnel: [_ w765] -> w742
              tunnel: [_ w764] -> w741
              tunnel: [_ w763] -> w740
              tunnel: [_ w762] -> w739
              tunnel: w738 -> [_ w761]
              tunnel: [_ w760] -> w737
              tunnel: [_ w759] -> w736
              tunnel: [_ w758] -> w735
              tunnel: [_ w757] -> w734
              tunnel: w733 -> [_ w756]
              tunnel: [_ w755] -> w732
              tunnel: w731 -> [_ w754]
              tunnel: w730 -> [_ w753]
              tunnel: [_ w752] -> w729
              tunnel: [_ 4] -> w728
              tunnel: w726 -> [w748 w750]
              tunnel: [w748 w749] -> w725
              frame Default {
              }
              frame "Logic" {
                n210 = for {
                  tunnel: [1.0 ("y")] -> w766 mode=indexing if=w772
                  tunnel: [0.0] -> w767 mode=indexing if=w772
                  tunnel: [2] -> w768 mode=indexing if=w772
                  tunnel: [w790] -> w769 mode=indexing if=w772
                  tunnel: [w789] -> w770 mode=indexing if=w772
                  tunnel: ["L" ("format string")] -> w765 mode=indexing if=w772
                  tunnel: [w777] -> w762 mode=indexing if=w772
                  tunnel: [w796] -> w764 mode=indexing if=w772
                  tunnel: [""] -> w763 mode=indexing if=w772
                  tunnel: [w794] -> w760 mode=indexing if=w772
                  tunnel: [w796] -> _ mode=indexing if=w772
                  tunnel: [w783] -> w759 mode=indexing if=w772
                  tunnel: w761 -> [w800]
                  tunnel: ["" ("format string")] -> w758 mode=indexing if=w772
                  tunnel: [w794] -> w757 mode=indexing if=w772
                  tunnel: w756 -> [w793]
                  tunnel: [i64 0] -> w755 mode=indexing if=w772
                  tunnel: w754 -> [w789] mode=indexing
                  tunnel: w753 -> [w775]
                  tunnel: [w773] -> w752 mode=indexing if=w772
                  tunnel: w750 -> [w771]
                  tunnel: [w771] -> w749
                  i -> [w794]
                  w772 = TRUE ("x != 0?")
                  n211 = Increment(x=w794) -> (x+1=w799:i32)
                  n212 = Format Into String(format string="Logic%d" ("KEY1"), w799) -> (resulting string=w773:string)  [unwired: 2 in, 1 out]
                  n213 = call "SearchKey.vi"("In"=w793, "KEY1"=w800, "KEY2"=w773) -> ("Data"=w802:string[])  [unwired: 12 out]
                  n214 = call "SearchKey.vi"("KEY1"=w775, "KEY2"=w773) -> ()  [unwired: 1 in, 13 out]
                  n215 = Index Array(array=w802, index #2=0 ("index")) -> (element #1=w777:string, element #3=w782:string, element #4=w781:string, element #5=w780:string)  [unwired: 4 in, 1 out]
                  n216 = Format Into String(format string="Logic%d %s" ("KEY1"), w799, w773) -> (resulting string=w796:string)  [unwired: 2 in, 1 out]
                  n217 = Bundle("0", w782, w781, w780) -> (w779:cluster{string, string, string, string})  [unwired: 1 in]
                  n218 = Decimal String To Number(string=w779, default (0L)=u8 0 ("index")) -> (number=w786:cluster{u8, u8, u8, u8})  [unwired: 1 in, 1 out]
                  n219 = Add(x=w789, y=100.0) -> (x+y=w790:dbl)
                  n220 = expression code="C*8"(w786) -> (w784:cluster{u8, u8, u8, u8})
                  n221 = Type Cast(type=u32 0 ("Color"), x=w784) -> (*(type *) &x=w783:u32)
                }
              }
            }
          }
          frame True {
            n222 = case shown="\"Logic\"" w806 {
              tunnel: [_ 1] -> w809
              tunnel: [_ i32[] [2]] -> w808
              tunnel: [_ i32[] [4]] -> w807
              frame Default {
              }
              frame "Logic" {
              }
            }
          }
        }
      }
      frame "Alarm" {
        n223 = case shown="TRUE" w815 {
          tunnel: [_ w836] -> w822
          tunnel: [_ w835] -> w821
          tunnel: [i32[] [10] w834] -> w820
          tunnel: w819 -> [_ w833]
          tunnel: [_ w832] -> w818
          tunnel: w815 -> [_ _]
          tunnel: [i32[] [2] w829] -> w817
          tunnel: [1 w828] -> w816
          tunnel: w814 -> [w823 w827]
          tunnel: [w823 w827] -> w813
          frame True {
          }
          frame False {
            n224 = for {
              N: 8 -> [_]
              tunnel: [1.0 ("y")] -> w835 mode=indexing if=w837
              tunnel: [0.0] -> w836 mode=indexing if=w837
              tunnel: [2] -> w829 mode=indexing if=w837
              tunnel: "$Amp" ("KEY1") -> [w849]
              tunnel: [w845] -> w834 mode=indexing if=w837
              tunnel: w833 -> [w844]
              tunnel: [1] -> w832 mode=indexing if=w837
              i -> [w845]
              n225 = Increment(x=w845) -> (x+1=w848:i32)
              n226 = Format Into String(format string="CH%d" ("KEY1"), w848) -> (resulting string=w850:string)  [unwired: 2 in, 1 out]
              n227 = call "SearchKey.vi"("In"=w844, "KEY1"=w849, "KEY2"=w850) -> ("Data"=w852:string[])  [unwired: 12 out]
              n228 = Index Array(array=w852, index=1) -> (element=w842:string)
              n229 = To Upper Case(1:w842) -> (0:w839:string)
              n230 = Not Equal?(x=w839, y=string[] ["OFF", "NC"]) -> (x != y?=w840:bool[])
              n231 = And Array Elements(Boolean array=w840) -> (logical AND=w837:bool)
            }
            n232 = Array Size(array=w829) -> (size(s)=w828:i32)
          }
        }
      }
      frame "AlarmLP", "AlarmLPL" {
        n233 = case shown="FALSE" w855 {
          tunnel: [w871 _] -> w863
          tunnel: [w870 _] -> w862
          tunnel: [w869 w907] -> w861
          tunnel: w860 -> [w868 _]
          tunnel: [w867 _] -> w859
          tunnel: w858 -> [w866 w906]
          tunnel: [w865 w909] -> w857
          tunnel: [w864 w908] -> w856
          frame False {
            n234 = case shown="\"Pulse\"" w866 {
              tunnel: [w878 _ w899] -> w865
              tunnel: [w875 _ w898] -> w871
              tunnel: [w874 _ w897] -> w870
              tunnel: [w877 _ w896] -> w869
              tunnel: w868 -> [w873 _ _]
              tunnel: [w876 _ w895] -> w867
              frame "Pulse" {
                n235 = for {
                  N: 4 -> [_]
                  tunnel: [1.0 ("y")] -> w874 mode=indexing if=w880
                  tunnel: [0.0] -> w875 mode=indexing if=w880
                  tunnel: [2] -> w878 mode=indexing if=w880
                  tunnel: "$Pulse" ("KEY1") -> [w889]
                  tunnel: [w883] -> w877 mode=indexing if=w880
                  tunnel: w873 -> [w882]
                  tunnel: [1] -> w876 mode=indexing if=w880
                  i -> [w883]
                  n236 = Increment(x=w883) -> (x+1=w888:i32)
                  n237 = Format Into String(format string="Pulse%d" ("KEY1"), w888) -> (resulting string=w890:string)  [unwired: 2 in, 1 out]
                  n238 = call "SearchKey.vi"("In"=w882, "KEY1"=w889, "KEY2"=w890) -> ("Data"=w892:string[])  [unwired: 12 out]
                  n239 = Index Array(array=w892) -> (element=w885:string)  [unwired: 1 in]
                  n240 = Not Equal?(x=w885, y="OFF") -> (x != y?=w880:bool)
                }
              }
              frame Default {
              }
              frame "Logic" {
                n241 = for {
                  N: 4 -> [_]
                  tunnel: [1.0 ("y")] -> w897 mode=indexing if=w900
                  tunnel: [0.0] -> w898 mode=indexing if=w900
                  tunnel: [2] -> w899 mode=indexing if=w900
                  tunnel: [w902] -> w896 mode=indexing if=w900
                  tunnel: [1] -> w895 mode=indexing if=w900
                  i -> [w902]
                  w900 = TRUE ("x != y?")
                }
              }
            }
            n242 = Array Size(array=w865) -> (size(s)=w864:i32)
          }
          frame True {
            n243 = case shown="デフォルト" w906 {
              tunnel: [_ i32[] [2]] -> w909
              tunnel: [_ 1] -> w908
              tunnel: [_ i32[] [4]] -> w907
              frame Default {
              }
              frame "Logic", "Pulse" {
              }
            }
          }
        }
      }
      frame "AlarmOut" {
        n244 = case shown="FALSE" w914 {
          tunnel: [w926 i32[] [2]] -> w920
          tunnel: [w925 _] -> w919
          tunnel: [w924 _] -> w918
          tunnel: [w923 i32[] [4]] -> w917
          tunnel: [w922 _] -> w916
          tunnel: [w921 1] -> w915
          frame False {
            w921 = 4
            n245 = for {
              N: w921 -> [_]
              tunnel: [1.0 ("y")] -> w924 mode=indexing
              tunnel: [0.0] -> w925 mode=indexing
              tunnel: [2] -> w926 mode=indexing
              tunnel: [w928] -> w923 mode=indexing
              tunnel: [1] -> w922 mode=indexing
              i -> [w928]
            }
          }
          frame True {
          }
        }
      }
    }
    n246 = expression code="N*2"(w224) -> (w228:i32)
    n247 = Initialize Array(w228, w226) -> (w227:i32[])
  }
  "ActiveCH" <- w2
  n248 = call "UnitConv(Time).vi"("St IN"=w32) -> ("NumOUT"=w19:dbl)  [unwired: 3 in, 5 out]
  n249 = Bundle(0, w85) -> (w52:cluster{i32, i16})  [unwired: 1 in]
  n250 = Add Array Elements(numeric array=w55) -> ()  [unwired: 1 out]
  n251 = Merge Errors(w20) -> (→"error out":errorcluster)
  n252 = Sort 1D Array(array=w74) -> (sorted array=w73:cluster{timestamp, i32}[])
  n253 = for {
    tunnel: w73 -> [w953] mode=indexing
    tunnel: [w944] -> w72 mode=indexing
    tunnel: w71 -> [w952]
    tunnel: w70 -> [w949]
    tunnel: w69 -> [w950]
    tunnel: w68 -> [w951]
    tunnel: [w948] -> w67 mode=indexing
    tunnel: [w947] -> w66 mode=indexing
    tunnel: [w937] -> w65 mode=indexing
    tunnel: [w938] -> w64 mode=indexing
    tunnel: w61 -> [w946]
    tunnel: [w945] -> w60 mode=indexing
    tunnel: w27 -> [w942]
    tunnel: [w936] -> w28 mode=indexing
    tunnel: w19 -> [w939]
    n254 = Unbundle(w953) -> (w944:timestamp, w943:i32)
    n255 = Index Array(array=w946, index=w943) -> (element=w945:refnum<file>)
    n256 = Index Array(array=w949, index=w943) -> (element=w947:refnum<file>)
    n257 = Index Array(array=w952, index=w943) -> (element=w948:timestamp)
    n258 = Index Array(array=w950, index=w943) -> ()  [unwired: 1 out]
    n259 = Index Array(array=w951, index=w943) -> (element=w938:i32)
    n260 = Index Array(array=w942, index=w943) -> (element=w941:i32)
    n261 = Multiply(x=w941, y=w939) -> (x*y=w940:dbl)
    n262 = Multiply(x=w938, y=w939) -> (x*y=w935:dbl)
    n263 = Subtract(x=w944, y=w940) -> (x-y=w936:timestamp)
    n264 = Add(x=w936, y=w935) -> (x+y=w937:timestamp)
  }
  n265 = call "UnitConv(Time).vi"("Num IN"=w19) -> ("St OUT"=w17:string)  [unwired: 3 in, 5 out]
  n266 = Build Array (concatenate)("<GBD>" ("element"), w17, w18) -> (→"Linkcheck":string[])
  n267 = Bundle By Name(cluster=T1 {"File"=[], "Idx"=[], "dT"=0.0, "Hd"=0, "Rd"=0, "Start"=[], "Trig"=[], "Stop"=[], "FirstPos"=[], "Count"=[], "Color"=[], "Label"=[], "INP"=[], "H"=[], "L"=[], "Fmt"=[], "Unit"=[], "SEL"=[], "Byte"=[], "Pos"=[], "Bit"=[], "Flg"=[], "Gain"=[], "Offset"=[], "CH"=[], "Opt"={"Mode"=0, "TUNIT"=enum."CELS"}, "TYPE"=enum."GBD", "Comp"=[], "Temp"=[]} ("Param"), "Comp"=w60, "File"=w66, "Hd"=w96, "Start"=w67, "Trig"=w72, "Stop"=w65, "Count"=w64, "FirstPos"=w28, "dT"=w19, "Rd"=w9, "L"=w54, "H"=w53, "Byte"=w81, "Pos"=w5, "Bit"=w51, "Flg"=w47, "Offset"=w80, "Gain"=w79, "CH"=w58, "Unit"=w56, "Fmt"=w78, "Label"=w37, "INP"=w63, "Color"=w57, "Temp"=w26, "Opt"=w52) -> (w45:T1)
  n268 = Unbundle By Name(w45) -> ("Label"=w44:string[])
  n269 = Build Array (concatenate)("Info", w37) -> (w36:string[])
  n270 = Build Array (concatenate)(w41, w40) -> (w35:string[])
  n271 = Build Array(w36, w35) -> (w34:string[][])
  n272 = Array Size(array=w44) -> (size(s)=w43:i32)
  n273 = Transpose 2D Array(2D array=w34) -> (transposed array=→"List":string[][])
  n274 = for {
    N: w43 -> [_]
    tunnel: [w954] -> w42 mode=indexing
    i -> [w954]
  }
  n275 = Bundle By Name(cluster=w45, "SEL"=w42) -> (→"Param":T1)
